vi "Update Controller State.vi"(8 "error in (no error)":errorcluster, 10 "Car Wash Controller State":T1, 11 "Car Wash Controller in":refnum<class "Car Wash Controller.lvclass">) -> (0 "error out":errorcluster, 3 "Car Wash Controller out":refnum<class "Car Wash Controller.lvclass">)   [LabVIEW 2012, in "Car Wash Controller.lvlib" / "Car Wash Controller.lvclass"]
uses:
  Car Wash Controller.lvclass
  Entry Console API/Entry Console API/Entry Console API.lvclass
  Wash Display Console API/Wash Display Console API/Wash Display Console API.lvclass
  Car Wash Controller State.ctl
  Vehical Position Interface API/Vehical Position Interface API/Vehicle Position Interface API.lvclass
  Configuration Database API/Configuration Database API/Configuration Database API.lvclass
  Vehicle Position.ctl
  Wash Step.ctl
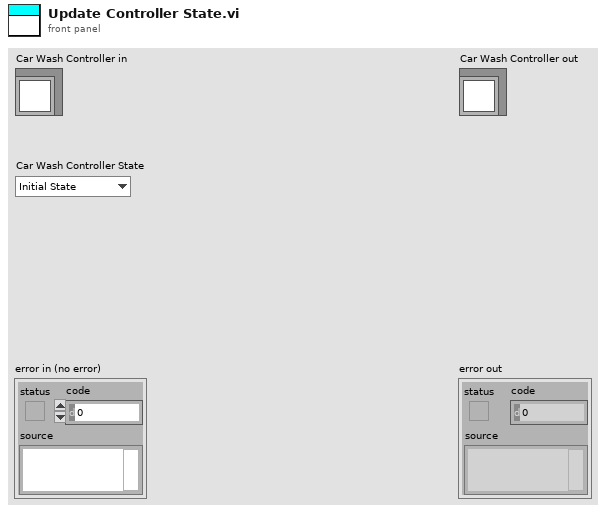
[diagram p1: front panel]
types:
  T1 = typedef "Car Wash Controller.lvlib/Car Wash Controller.lvclass/Car Wash Controller State.ctl" = enum16{"Initial State", "Wait For Start State", "Start State", "Wait For Vehicle Position State", "Wash Step Execution State", "Wash Step / Cycle Completion State", "Wash Exit State", "Wash Abort / Terminate State"}
  T2 = typedef "Car Wash Controller.lvlib/Car Wash Controller.lvclass/Vehicle Position.ctl" = enum16{"Entry", "Station 1", "Station 2", "Station 3", "Exit"}
  T3 = typedef "Car Wash Controller.lvlib/Car Wash Controller.lvclass/Wash Step.ctl" = enum16{"Under Body Wash", "Bug Remover", "Pre-Soak", "High Pressure Wash", "Low Pressure Wax", "Spot Free Rince", "Tire Shine Foam", "Air Dry"}
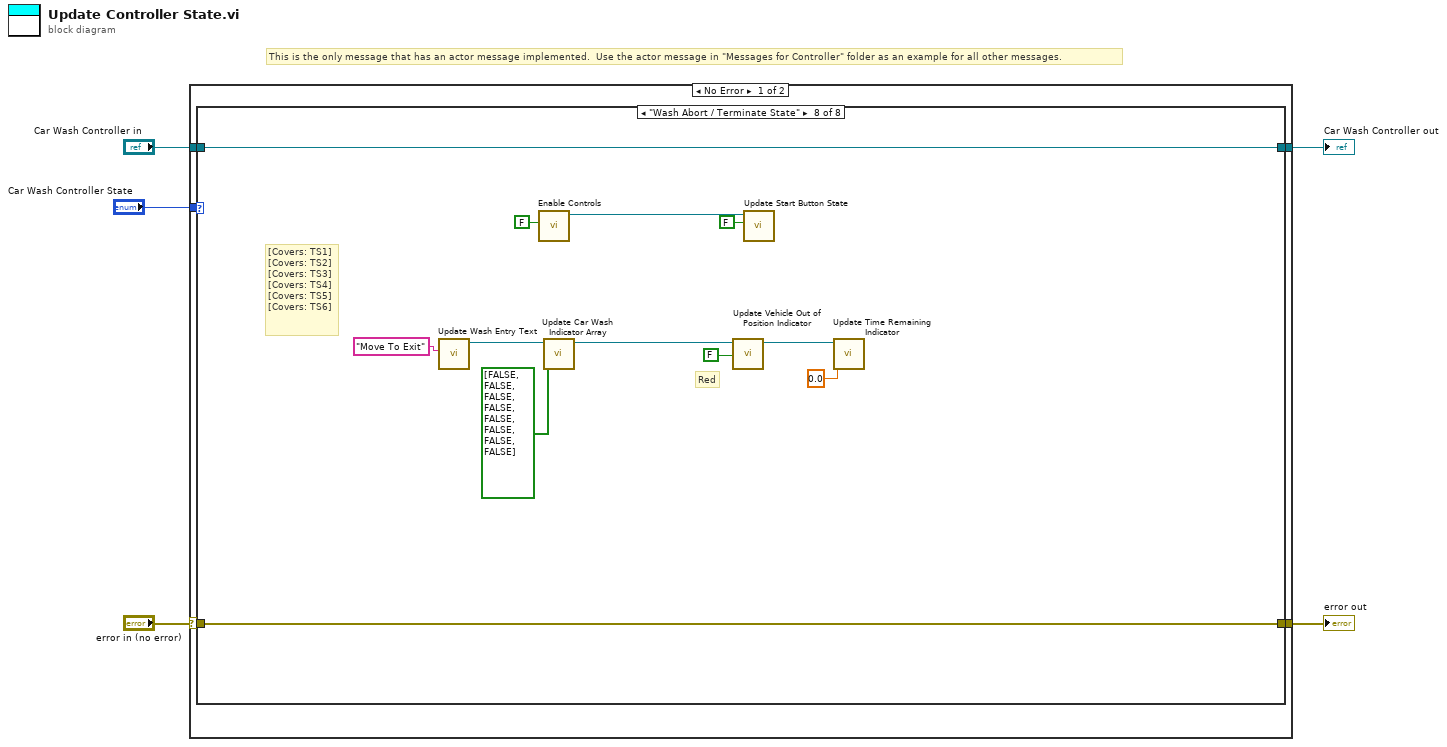
[diagram p0: block diagram]
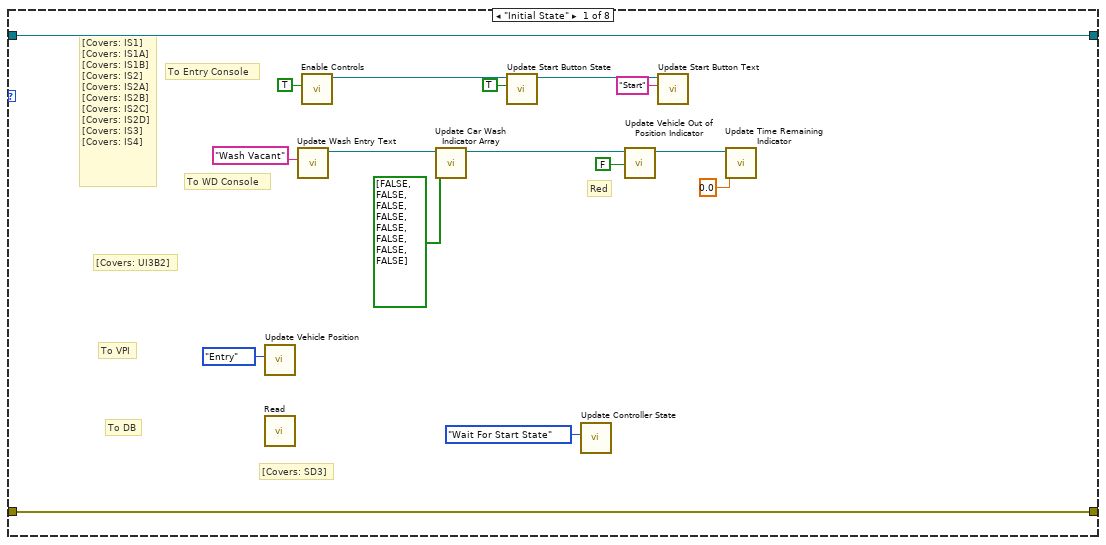
[diagram p2: hidden frame]
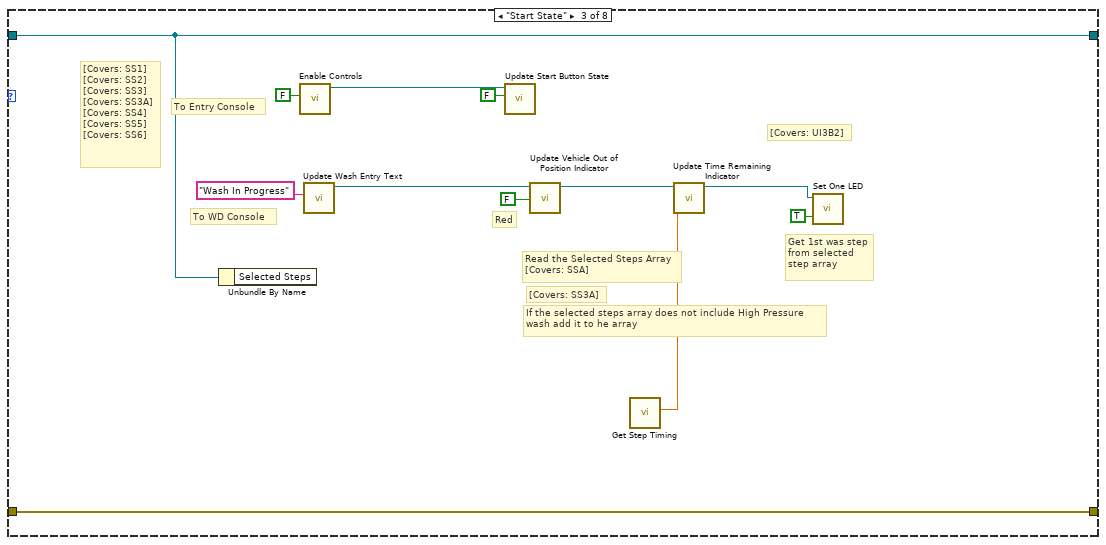
[diagram p4: hidden frame]
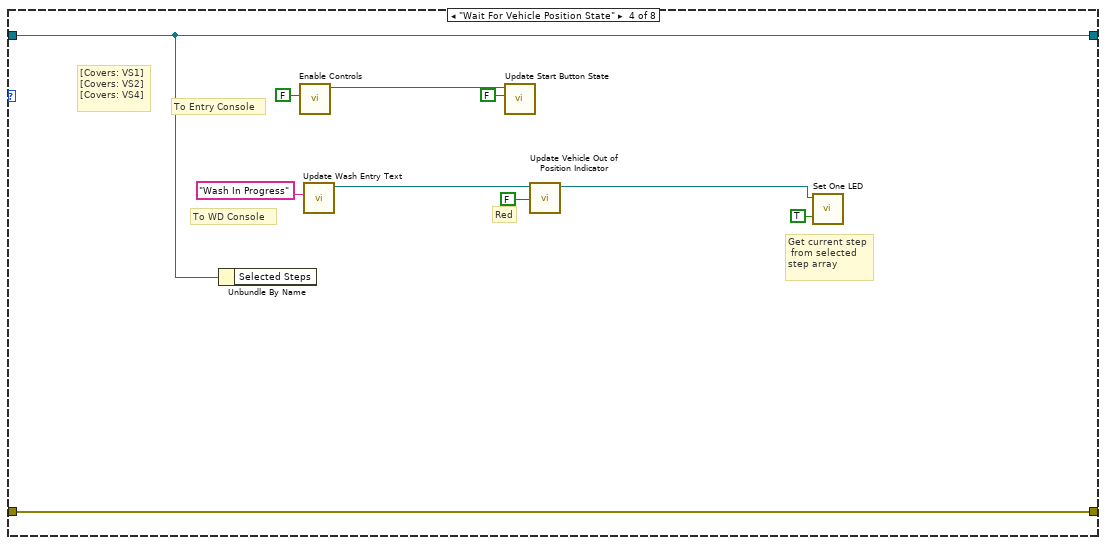
[diagram p5: hidden frame]
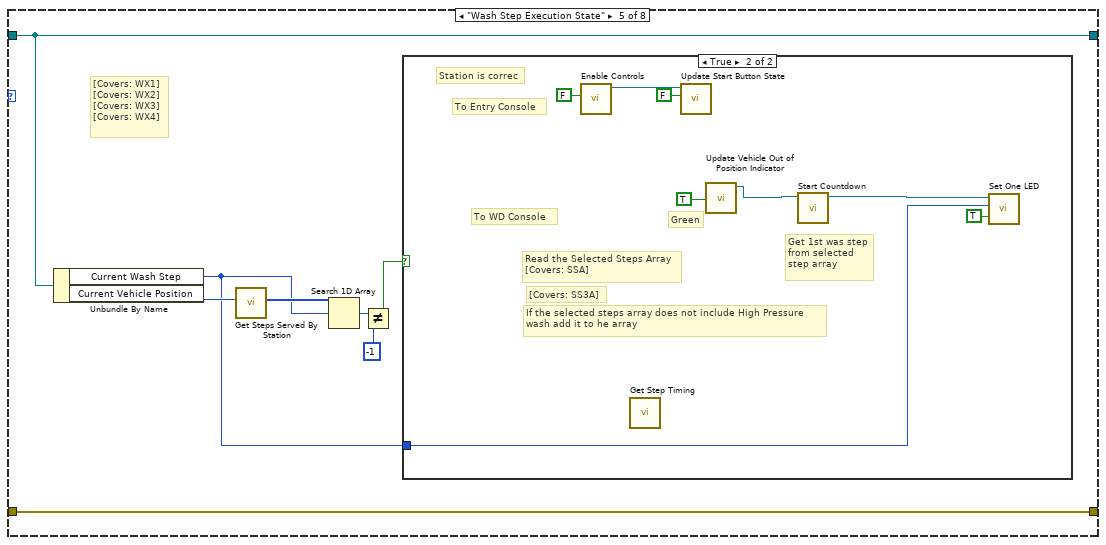
[diagram p6: hidden frame]
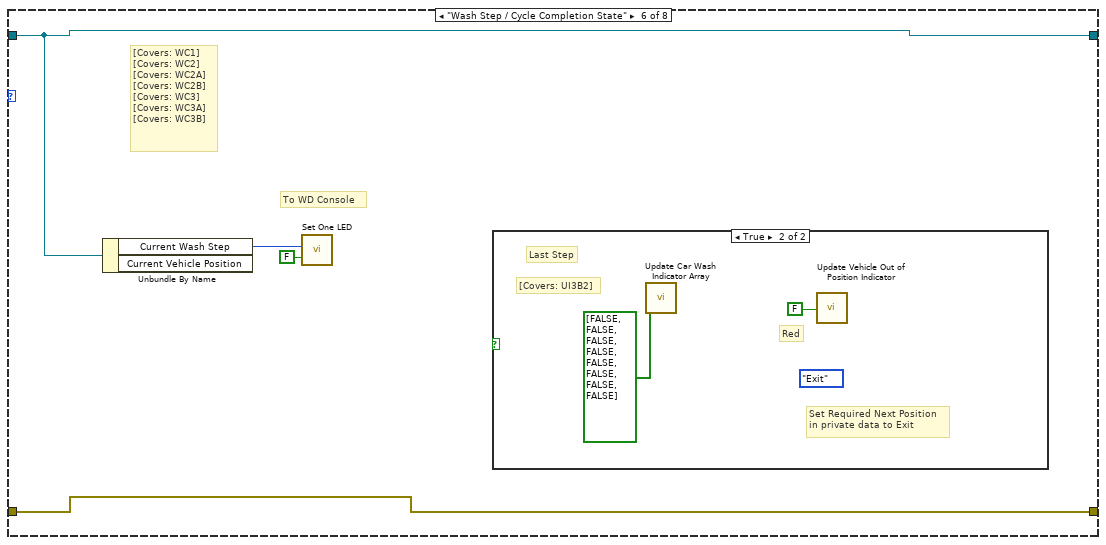
[diagram p8: hidden frame]
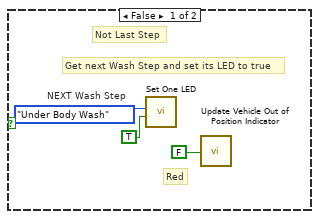
[diagram p9: hidden frame]
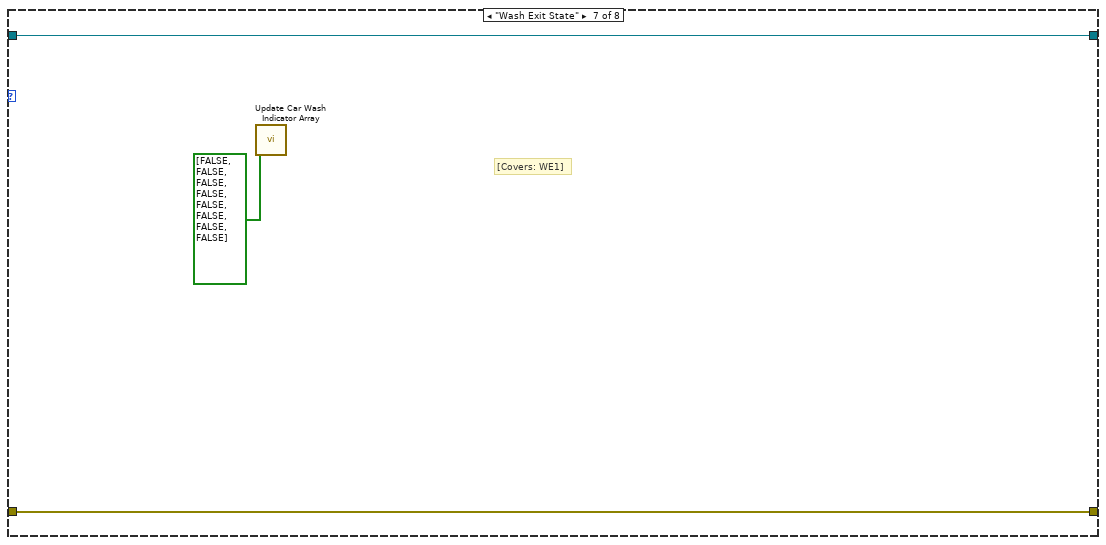
[diagram p10: hidden frame]
diagram:
  # "This is the only message that has an actor message implemented.  Use the actor message in \"Messages for Controller\" folder as an example for all other messages."
  n1 = case shown="No Error" "error in (no error)" {
    selector: "error in (no error)" -> [w8 w92]
    tunnel: [w7 w92] -> w4
    tunnel: [w9 w91] -> w2
    tunnel: "Car Wash Controller in" -> [w10 w91]
    tunnel: "Car Wash Controller State" -> [w6 _]
    frame No Error {
      n2 = case shown="\"Wash Abort / Terminate State\"" w6 {
        tunnel: [w13 w28 w30 w43 w57 w69 w78 w90] -> w9
        tunnel: w10 -> [w13 w28 w30 w43 w57 w69 w78 w90]
        tunnel: [w12 w27 w40 w50 w58 w70 w77 w89] -> w7
        tunnel: w8 -> [w12 w27 w40 w50 w58 w70 w77 w89]
        frame "Initial State" {
          # "[Covers: SD3]"
          # "[Covers: UI3B2]"
          # "Red"
          # "To VPI"
          # "To WD Console"
          # "To DB"
          # "[Covers: IS1]\n[Covers: IS1A]\n[Covers: IS1B]\n[Covers: IS2]\n[Covers: IS2A]\n[Covers: IS2B]\n[Covers: IS2C]\n[Covers: IS2D]\n[Covers: IS3]\n[Covers: IS4]"
          # "To Entry Console"
          n3 = call-dynamic "Update Vehicle Position.vi"("Vehicle Position"=Vehicle_Position."Entry") -> ()  [unwired: 9 in, 2 out]
          n4 = call-dynamic "Read.vi"() -> ()  [unwired: 10 in, 2 out]
          n5 = call-dynamic "Update Wash Entry Text.vi"("Wash Entry Text"="Wash Vacant") -> ("Wash Display Console API out"=w20:refnum<class "Wash Display Console API.lvclass">)  [unwired: 9 in, 1 out]
          n6 = call-dynamic "Enable Controls.vi"("Controls"=TRUE) -> ("Entry Console API out"=w26:refnum<class "Entry Console API.lvclass">)  [unwired: 9 in, 1 out]
          n7 = call-dynamic "Update Car Wash Indicator Array.vi"("Car Wash Indicator Array"=bool[] [FALSE, FALSE, FALSE, FALSE, FALSE, FALSE, FALSE, FALSE], "Wash Display Console API in"=w20) -> ("Wash Display Console API out"=w19:refnum<class "Wash Display Console API.lvclass">)  [unwired: 8 in, 1 out]
          n8 = call-dynamic "Update Start Button State.vi"("Start Button State"=TRUE ("Start Button"), "Entry Console API in"=w26) -> ("Entry Console API out"=w25:refnum<class "Entry Console API.lvclass">)  [unwired: 8 in, 1 out]
          n9 = call "Update Controller State.vi"("Car Wash Controller State"=Car_Wash_Controller_State."Wait For Start State") -> ()  [unwired: 9 in, 2 out]
          n10 = call-dynamic "Update Vehicle Out of Position Indicator.vi"("Vehicle Out of Pos"=FALSE, "Wash Display Console API in"=w19) -> ("Wash Display Console API out"=w18:refnum<class "Wash Display Console API.lvclass">)  [unwired: 8 in, 1 out]
          n11 = call-dynamic "Update Start Button Text.vi"("Start Button Text"="Start", "Entry Console API in"=w25) -> ()  [unwired: 8 in, 2 out]
          n12 = call-dynamic "Update Time Remaining Indicator.vi"("Time Remaining"=0.0, "Wash Display Console API in"=w18) -> ()  [unwired: 8 in, 2 out]
        }
        frame "Wait For Start State" {
          # "[Covers: WS1]\n[Covers: WS3]"
        }
        frame "Start State" {
          # "[Covers: UI3B2]"
          # "Get 1st was step\nfrom selected\nstep array"
          # "[Covers: SS1]\n[Covers: SS2]\n[Covers: SS3]\n[Covers: SS3A]\n[Covers: SS4]\n[Covers: SS5]\n[Covers: SS6]"
          # "Red"
          # "Read the Selected Steps Array\n[Covers: SSA]"
          # "[Covers: SS3A]"
          # "If the selected steps array does not include High Pressure\nwash add it to he array"
          # "To WD Console"
          # "To Entry Console"
          n13 = Unbundle By Name(w30) -> ()  [unwired: 1 out]
          n14 = call-dynamic "Enable Controls.vi"("Controls"=FALSE) -> ("Entry Console API out"=w34:refnum<class "Entry Console API.lvclass">)  [unwired: 9 in, 1 out]
          n15 = call-dynamic "Update Wash Entry Text.vi"("Wash Entry Text"="Wash In Progress") -> ("Wash Display Console API out"=w29:refnum<class "Wash Display Console API.lvclass">)  [unwired: 9 in, 1 out]
          n16 = call-dynamic "Update Start Button State.vi"("Start Button State"=FALSE ("Start Button"), "Entry Console API in"=w34) -> ()  [unwired: 8 in, 2 out]
          n17 = call-dynamic "Update Vehicle Out of Position Indicator.vi"("Vehicle Out of Pos"=FALSE, "Wash Display Console API in"=w29) -> ("Wash Display Console API out"=w38:refnum<class "Wash Display Console API.lvclass">)  [unwired: 8 in, 1 out]
          n18 = call "Get Step Timing.vi"() -> ("Step Timing"=w33:dbl)  [unwired: 9 in, 2 out]
          n19 = call-dynamic "Update Time Remaining Indicator.vi"("Time Remaining"=w33, "Wash Display Console API in"=w38) -> ("Wash Display Console API out"=w32:refnum<class "Wash Display Console API.lvclass">)  [unwired: 8 in, 1 out]
          n20 = call-dynamic "Set One LED.vi"("Value"=TRUE, "Wash Display Console API in"=w32) -> ()  [unwired: 8 in, 2 out]
        }
        frame "Wait For Vehicle Position State" {
          # "[Covers: VS1]\n[Covers: VS2]\n[Covers: VS4]"
          # "Get current step\n from selected\nstep array"
          # "Red"
          # "To WD Console"
          # "To Entry Console"
          n21 = Unbundle By Name(w43) -> ()  [unwired: 1 out]
          n22 = call-dynamic "Enable Controls.vi"("Controls"=FALSE) -> ("Entry Console API out"=w45:refnum<class "Entry Console API.lvclass">)  [unwired: 9 in, 1 out]
          n23 = call-dynamic "Update Wash Entry Text.vi"("Wash Entry Text"="Wash In Progress") -> ("Wash Display Console API out"=w42:refnum<class "Wash Display Console API.lvclass">)  [unwired: 9 in, 1 out]
          n24 = call-dynamic "Update Start Button State.vi"("Start Button State"=FALSE ("Start Button"), "Entry Console API in"=w45) -> ()  [unwired: 8 in, 2 out]
          n25 = call-dynamic "Update Vehicle Out of Position Indicator.vi"("Vehicle Out of Pos"=FALSE, "Wash Display Console API in"=w42) -> ("Wash Display Console API out"=w41:refnum<class "Wash Display Console API.lvclass">)  [unwired: 8 in, 1 out]
          n26 = call-dynamic "Set One LED.vi"("Value"=TRUE, "Wash Display Console API in"=w41) -> ()  [unwired: 8 in, 2 out]
        }
        frame "Wash Step Execution State" {
          # "[Covers: WX1]\n[Covers: WX2]\n[Covers: WX3]\n[Covers: WX4]"
          n27 = Unbundle By Name(w57) -> ("Current Wash Step"=w51:T3, "Current Vehicle Position"=w56:T2)
          n28 = call "Get Steps Served By Station.vi"("Vehicle Position"=w56) -> ("Steps Served By Station"=w55:T3[])  [unwired: 8 in, 2 out]
          n29 = Search 1D Array(1D array=w55, element=w51) -> (index of element=w54:i32)  [unwired: 1 in]
          n30 = Not Equal?(x=w54, y=-1) -> (x != y?=w52:bool)
          n31 = case shown="True" w52 {
            tunnel: w51 -> [_ w61]
            frame False {
              # "Car is not in correct station do nothing."
            }
            frame True {
              # "Station is correc"
              # "Get 1st was step\nfrom selected\nstep array"
              # "Green"
              # "Read the Selected Steps Array\n[Covers: SSA]"
              # "[Covers: SS3A]"
              # "If the selected steps array does not include High Pressure\nwash add it to he array"
              # "To WD Console"
              # "To Entry Console"
              n32 = call-dynamic "Enable Controls.vi"("Controls"=FALSE) -> ("Entry Console API out"=w63:refnum<class "Entry Console API.lvclass">)  [unwired: 9 in, 1 out]
              n33 = call "Get Step Timing.vi"() -> ()  [unwired: 9 in, 3 out]
              n34 = call-dynamic "Update Start Button State.vi"("Start Button State"=FALSE ("Start Button"), "Entry Console API in"=w63) -> ()  [unwired: 8 in, 2 out]
              n35 = call-dynamic "Update Vehicle Out of Position Indicator.vi"("Vehicle Out of Pos"=TRUE) -> ("Wash Display Console API out"=w60:refnum<class "Wash Display Console API.lvclass">)  [unwired: 9 in, 1 out]
              n36 = call-dynamic "Start Countdown.vi"("Wash Display Console API in"=w60) -> ("Wash Display Console API out"=w59:refnum<class "Wash Display Console API.lvclass">)  [unwired: 9 in, 1 out]
              n37 = call-dynamic "Set One LED.vi"("Value"=TRUE, "Wash Step"=w61, "Wash Display Console API in"=w59) -> ()  [unwired: 7 in, 2 out]
            }
          }
        }
        frame "Wash Step / Cycle Completion State" {
          # "[Covers: WC1]\n[Covers: WC2]\n[Covers: WC2A]\n[Covers: WC2B]\n[Covers: WC3]\n[Covers: WC3A]\n[Covers: WC3B]"
          # "To WD Console"
          n38 = Unbundle By Name(w69) -> ("Current Wash Step"=w67:T3)  [unwired: 1 out]
          n39 = call-dynamic "Set One LED.vi"("Value"=FALSE, "Wash Step"=w67) -> ()  [unwired: 8 in, 2 out]
          n40 = case shown="True" {
            selector: _ -> [_ _]
            frame False {
              w71 = Wash_Step."Under Body Wash"  # NEXT Wash Step
              # "Get next Wash Step and set its LED to true"
              # "Red"
              # "Not Last Step"
              n41 = call-dynamic "Set One LED.vi"("Value"=TRUE, "Wash Step"=w71) -> ()  [unwired: 8 in, 2 out]
              n42 = call-dynamic "Update Vehicle Out of Position Indicator.vi"("Vehicle Out of Pos"=FALSE) -> ()  [unwired: 9 in, 2 out]
            }
            frame True {
              (unwired) Vehicle_Position."Exit" ("Vehicle Position")
              # "[Covers: UI3B2]"
              # "Set Required Next Position\nin private data to Exit"
              # "Red"
              # "Last Step"
              n43 = call-dynamic "Update Car Wash Indicator Array.vi"("Car Wash Indicator Array"=bool[] [FALSE, FALSE, FALSE, FALSE, FALSE, FALSE, FALSE, FALSE]) -> ()  [unwired: 9 in, 2 out]
              n44 = call-dynamic "Update Vehicle Out of Position Indicator.vi"("Vehicle Out of Pos"=FALSE) -> ()  [unwired: 9 in, 2 out]
            }
          }
        }
        frame "Wash Exit State" {
          # "[Covers: WE1]"
          n45 = call-dynamic "Update Car Wash Indicator Array.vi"("Car Wash Indicator Array"=bool[] [FALSE, FALSE, FALSE, FALSE, FALSE, FALSE, FALSE, FALSE]) -> ()  [unwired: 9 in, 2 out]
        }
        frame "Wash Abort / Terminate State" {
          # "[Covers: TS1]\n[Covers: TS2]\n[Covers: TS3]\n[Covers: TS4]\n[Covers: TS5]\n[Covers: TS6]"
          # "Red"
          n46 = call-dynamic "Update Wash Entry Text.vi"("Wash Entry Text"="Move To Exit") -> ("Wash Display Console API out"=w80:refnum<class "Wash Display Console API.lvclass">)  [unwired: 9 in, 1 out]
          n47 = call-dynamic "Enable Controls.vi"("Controls"=FALSE) -> ("Entry Console API out"=w88:refnum<class "Entry Console API.lvclass">)  [unwired: 9 in, 1 out]
          n48 = call-dynamic "Update Car Wash Indicator Array.vi"("Car Wash Indicator Array"=bool[] [FALSE, FALSE, FALSE, FALSE, FALSE, FALSE, FALSE, FALSE], "Wash Display Console API in"=w80) -> ("Wash Display Console API out"=w85:refnum<class "Wash Display Console API.lvclass">)  [unwired: 8 in, 1 out]
          n49 = call-dynamic "Update Vehicle Out of Position Indicator.vi"("Vehicle Out of Pos"=FALSE, "Wash Display Console API in"=w85) -> ("Wash Display Console API out"=w84:refnum<class "Wash Display Console API.lvclass">)  [unwired: 8 in, 1 out]
          n50 = call-dynamic "Update Start Button State.vi"("Start Button State"=FALSE ("Start Button"), "Entry Console API in"=w88) -> ()  [unwired: 8 in, 2 out]
          n51 = call-dynamic "Update Time Remaining Indicator.vi"("Time Remaining"=0.0, "Wash Display Console API in"=w84) -> ()  [unwired: 8 in, 2 out]
        }
      }
    }
    frame Error {
    }
  }
  "error out" <- w4
  "Car Wash Controller out" <- w2
